vi "Digitize with Configuration (Single Point).vi"(8 "error in (no error)":errorcluster, 9 "Buffer Elements":u16(ring) items=["Date", "Extra", "Formatted", "Fractional", "Relative", "Seconds", "Status", "Time", "Timestamp", "Unit"], 10 "Buffer Name":string="defbuffer1", 11 "VISA resource name":refnum<visa-resource-name>) -> (0 "error out":errorcluster, 1 "Element Value":string, 2 "Digitize Value":dbl, 3 "VISA resource name out":refnum<visa-resource-name>)   [LabVIEW 2018, in "Keithley DMM7512.lvlib"]
doc: "This VI makes a digitize measurement using the specified function and stores the reading in a\nreading buffer and returns returns the last reading."
uses:
  <instrlib>/Keithley DMM7512/Keithley DMM7512.lvlib
panel:
  in  "Function":u16(ring) items=["Digitize Voltage", "Digitize Current"]
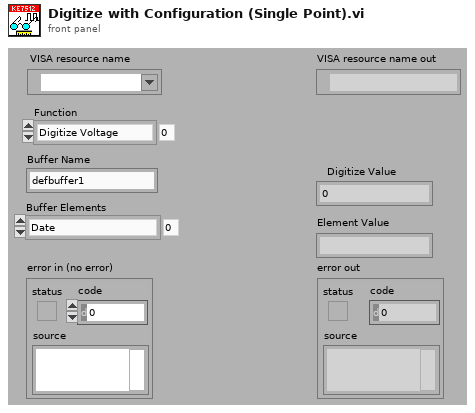
[diagram p1: front panel]
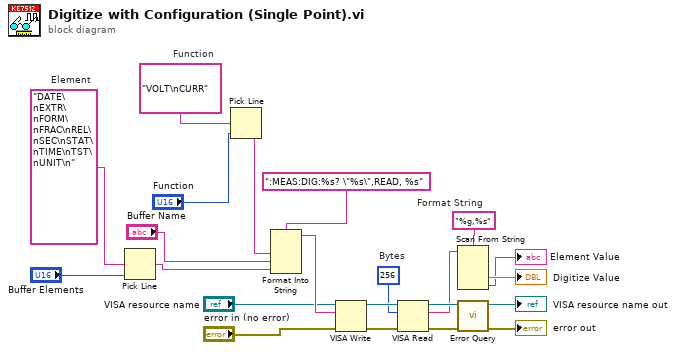
[diagram p0: block diagram]
diagram:
  w5 = "VOLT\nCURR"  # Function
  w8 = "DATE\nEXTR\nFORM\nFRAC\nREL\nSEC\nSTAT\nTIME\nTST\nUNIT\n"  # Element
  w14 = "%g,%s"  # Format String
  w20 = u32 256  # Bytes
  n1 = Pick Line(multi-line string=w8, line index="Buffer Elements") -> (output string=w1:string)  [unwired: 1 out]
  n2 = Pick Line(multi-line string=w5, line index="Function") -> (output string=w3:string)  [unwired: 1 out]
  n3 = Format Into String(format string=":MEAS:DIG:%s? \"%s\",READ, %s", w3, "Buffer Name", w1) -> (resulting string=w13:string)  [unwired: 2 in, 1 out]
  n4 = VISA Write(VISA resource name="VISA resource name", write buffer=w13, error in (no error)="error in (no error)") -> (VISA resource name out=w21:refnum<visa-resource-name>, error out=w22:errorcluster)  [unwired: 1 out]
  n5 = VISA Read(VISA resource name=w21, byte count=w20, error in (no error)=w22) -> (VISA resource name out=w19:refnum<visa-resource-name>, read buffer=w15:string, error out=w18:errorcluster)  [unwired: 1 out]
  n6 = Scan From String(format string=w14, input string=w15) -> (output 1=→"Digitize Value":dbl, output 2=→"Element Value":string)  [unwired: 4 in, 3 out]
  n7 = call <instrlib>:"Error Query.vi"("error in (no error)"=w18, "VISA resource name"=w19) -> ("error out"=→"error out":errorcluster, "VISA resource name out"=→"VISA resource name out":refnum<visa-resource-name>)  [unwired: 6 in, 2 out]
